vi "createDataFile.vi"(8 "error in (no error)":errorcluster, 11 "replace string (\"\")":string) -> (0 "error out":errorcluster, 2 "VI Name":string, 3 "Byte Stream File out":refnum<file>)   [LabVIEW 2019]
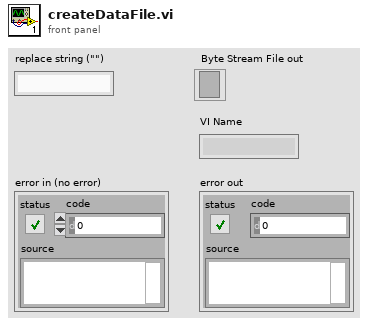
[diagram p1: front panel]
types:
  T1 = enum32{"invalid app kind", "Development System", "Run Time System", "Student Edition", "Embedded LabVIEW", "Evaluation", "Custom"}
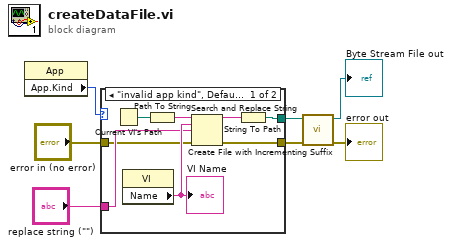
[diagram p0: block diagram]
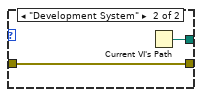
[diagram p2: hidden frame]
diagram:
  n1 = property class="App"() -> ("App.Kind"=w2:T1)  [unwired: 2 in, 2 out]
  n2 = case shown="\"invalid app kind\", Default" w2 {
    tunnel: [w15 w17] -> w3
    tunnel: "replace string (\"\")" -> [w10 _]
    tunnel: [w9 w16] -> w1
    tunnel: "error in (no error)" -> [w8 w16]
    frame "invalid app kind", Default {
      n3 = Current VI's Path() -> (path=w12:path)
      n4 = property class="VI"() -> ("Name"=w11:string)  [unwired: 2 in, 2 out]
      "VI Name" <- w11
      n5 = Path To String(path=w12) -> (string=w13:string)
      n6 = Search and Replace String(input string=w13, search string=w11, replace string=w10, error in=w8) -> (result string=w14:string, error out=w9:errorcluster)  [unwired: 4 in, 2 out]
      n7 = String To Path(string=w14) -> (path=w15:path)
    }
    frame "Development System" {
      n8 = Current VI's Path() -> (path=w17:path)
    }
  }
  n9 = call <vilib>:"Create File with Incrementing Suffix.vi"("error in (no error)"=w1, "file path"=w3) -> ("error out"=→"error out":errorcluster, "refnum out"=→"Byte Stream File out":refnum<file>)  [unwired: 7 in, 1 out]
